vi "core_RunningAllanInit.vi"(8 "error in (no error)":errorcluster, 11 "lengths":i32[](array[numeric])) -> (0 "error out":errorcluster, 3 "RACarry cluster":T1, 4 "histN":i32)   [LabVIEW 2015]
uses:
  core_RunningAllanCarry.vi
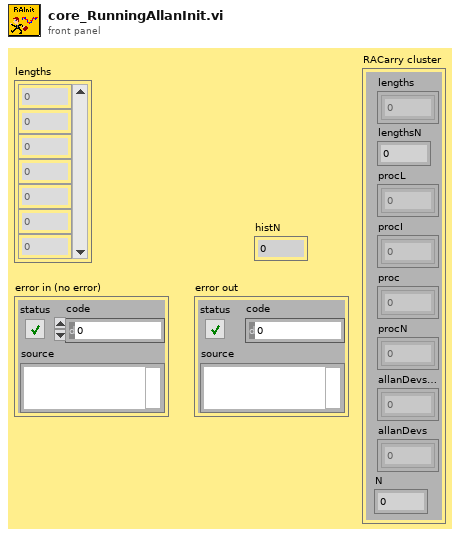
[diagram p1: front panel]
types:
  T1 = typedef "core_RunningAllanCarry.vi" = cluster{"lengths":i32[], "lengthsN":i32, "procL":i32[], "procI":i32[], "proc":dbl[], "procN":i32[], "allanDevsWIP":dbl[], "allanDevs":dbl[], "N":i32}
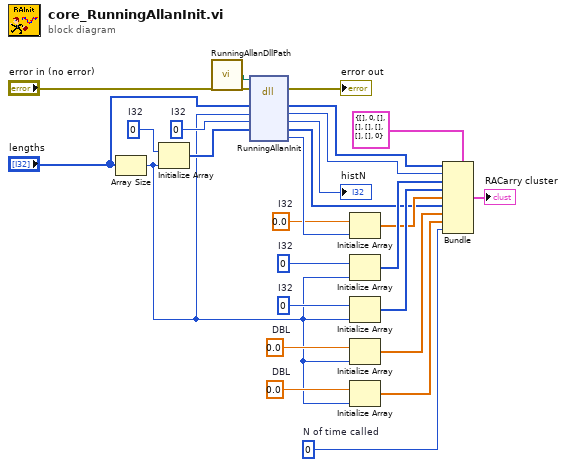
[diagram p0: block diagram]
diagram:
  w1 = 0  # N of time called
  w13 = 0.0  # DBL
  w14 = 0.0  # DBL
  w15 = 0  # I32
  w16 = 0  # I32
  w18 = 0.0  # I32
  w21 = 0  # I32
  w20 = 0  # I32
  n1 = Array Size(array="lengths") -> (size(s)=w12:i32)
  n2 = Initialize Array(w20, w12) -> (w22:i32[])
  n3 = call "RunningAllanDllPath.vi"() -> ("dll path"=w26:path)
  n4 = dll-call lib="C:/Users/srmgroup/CEAS v1/utils/average_tools/cores/RunningAllanCpp/RunningAllan.dll" fn="RunningAllanInit"(path in=w26, error in="error in (no error)", "lengths"="lengths", "lengthsN"=w12, "histN"=w21, "procN"=w22) -> (error out=→"error out":errorcluster, "lengths"=w10:i32[], "lengthsN"=w9:i32, "histN"=→"histN":i32, "procN"=w5:i32[], "procLength"=w19:i32)  [unwired: 3 in, 1 out]
  n5 = Initialize Array(w18, w19) -> (w6:dbl[])
  n6 = Initialize Array(w16, w12) -> (w8:i32[])
  n7 = Initialize Array(w15, w12) -> (w7:i32[])
  n8 = Initialize Array(w14, w12) -> (w4:dbl[])
  n9 = Initialize Array(w13, w12) -> (w3:dbl[])
  n10 = Bundle(cluster=T1 {"lengths"=[], "lengthsN"=0, "procL"=[], "procI"=[], "proc"=[], "procN"=[], "allanDevsWIP"=[], "allanDevs"=[], "N"=0}, "lengths"=w10, "lengthsN"=w9, "procL"=w8, "procI"=w7, "proc"=w6, "procN"=w5, "allanDevsWIP"=w4, "allanDevs"=w3, "N"=w1) -> (→"RACarry cluster":T1)
